vi "Set Bit.vi"(9 "value":bool, 10 "index mask":u8=2 format="%.0x", 11 "Byte in":u8 format="%.0x") -> (3 "Byte out":u8 format="%.0x")   [LabVIEW 2013]
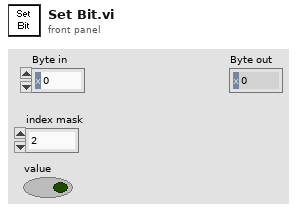
[diagram p1: front panel]
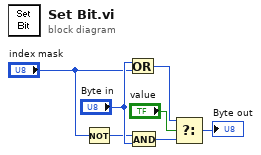
[diagram p0: block diagram]
diagram:
  n1 = Not(x="index mask") -> (.not. x?=w3:u8)
  n2 = Or(x="Byte in", y="index mask") -> (x .or. y?=w6:u8)
  n3 = And(x=w3, y="Byte in") -> (x .and. y?=w7:u8)
  n4 = Select(t=w6, s="value", f=w7) -> (s? t:f=→"Byte out":u8)
